vi "Create Pool.vi"(7 "FIFO Options":T1, 8 "error in (no error)":errorcluster, 10 "number of elements":u32, 11 "Pool type":refnum<class "Pool.lvclass">) -> (0 "error out":errorcluster, 3 "Pool":refnum<class "Pool.lvclass">)   [LabVIEW 2017, in "DSF Core.lvlib" / "Pool.lvclass"]
uses:
  Pool.lvclass
  Typedefs/DSF FIFO Options.ctl
  Pool.lvclass/Pool.ctl
  DSF Core.lvlib
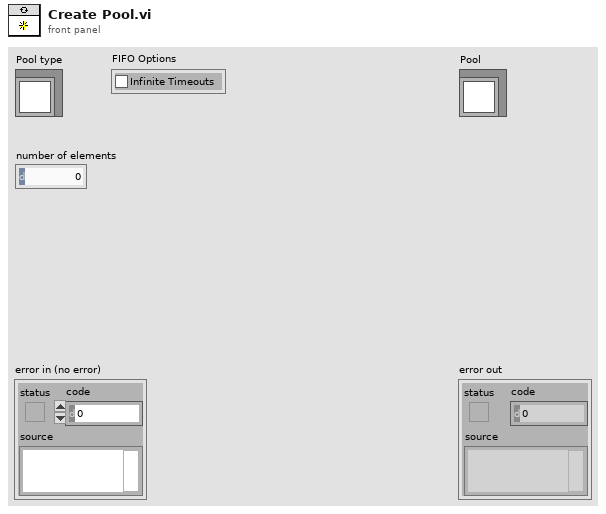
[diagram p1: front panel]
types:
  T1 = typedef "DSF Core.lvlib/DSF FIFO Options.ctl" = cluster{"Infinite Timeouts":bool}
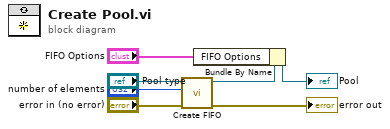
[diagram p0: block diagram]
diagram:
  n1 = call "Create FIFO.vi"("error in (no error)"="error in (no error)", "number of elements"="number of elements", "Pool in"="Pool type") -> ("error out"=→"error out":errorcluster, "Pool out"=w4:refnum<class "Pool.lvclass">)  [unwired: 7 in]
  n2 = Bundle By Name(cluster=w4, "FIFO Options"="FIFO Options") -> (→"Pool":refnum<class "Pool.lvclass">)
